vi "Initialize StartupBehavior Attribute.vi"(7 "Attribute.StartupBehavior in":refnum<class "Attribute.StartupBehavior.lvclass">, 11 "Behavior (Immediate)":T1) -> (3 "Attribute.StartupBehavior":refnum<class "Attribute.StartupBehavior.lvclass">)   [LabVIEW 2019, in "Attribute.StartupBehavior.lvclass"]
doc: "JKI State Machine Objects (SMO) 1.3.0.56\nJKI - JKI\nCopyright (c) 2017, JKI"
uses:
  Attribute.StartupBehavior.lvclass
  ProcessStartupBehavior.ctl
  Attribute.StartupBehavior.lvclass/Attribute.StartupBehavior.ctl
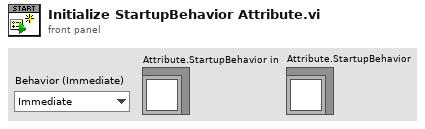
[diagram p1: front panel]
types:
  T1 = typedef "Attribute.StartupBehavior.lvclass/ProcessStartupBehavior.ctl" = enum16{"Immediate", "First Call", "Never"}
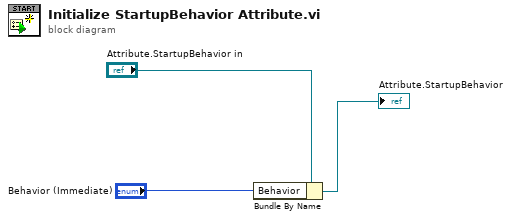
[diagram p0: block diagram]
diagram:
  n1 = Bundle By Name(cluster="Attribute.StartupBehavior in", "Behavior"="Behavior (Immediate)") -> (→"Attribute.StartupBehavior":refnum<class "Attribute.StartupBehavior.lvclass">)
